vi "Actor Core.vi"(8 "error in":errorcluster, 11 "TimeTracker in":refnum<class "TimeTracker.lvclass">) -> (0 "error out":errorcluster, 3 "Actor out":refnum<class "Actor.lvclass">)   [LabVIEW 2016, in "TimeTracker.lvclass"]
doc: "(<B>Filename</B>: Actor Framework.lvlib:Actor.lvclass:Actor Core.vi)\n\nReceives messages to the actor, reacts to them, and initiates any error handling that may shut the actor down.\n\nDescendant classes may override this VI to append parallel tasks for the actor to complete while it handles messages. Overrides use the Call Parent Method node."
uses:
  TimeTracker.lvclass
  C:/Program Files (x86)/National Instruments/LabVIEW 2016/vi.lib/ActorFramework/Actor/Actor.lvclass
  <vilib>/ActorFramework/Actor/Actor.lvclass
  <vilib>/Utility/miscctls.llb/LVRectTypeDef.ctl
  DisplayWindow/DisplayWindow/DisplayWindow/DisplayWindow.lvclass
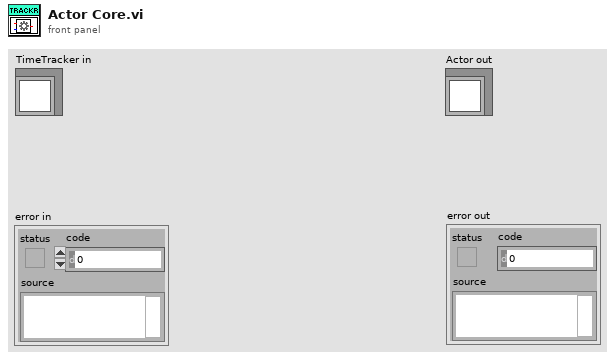
[diagram p1: front panel]
types:
  T1 = typedef "LVRectTypeDef.ctl" = cluster{"Left":i16, "Top":i16, "Right":i16, "Bottom":i16}
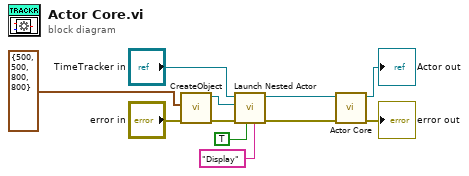
[diagram p0: block diagram]
diagram:
  n1 = call "CreateObject.vi"("error in (no error)"="error in", "Bounds"=T1 {"Left"=500, "Top"=500, "Right"=800, "Bottom"=800}) -> ("error out"=w1:errorcluster, "DisplayWindow out"=w4:refnum<class "DisplayWindow.lvclass">)  [unwired: 8 in]
  n2 = call <vilib>:"Launch Nested Actor.vi"("Debug Alias"="Display", "Open Actor Core front panel? (F)"=TRUE, "error in (no error)"=w1, "Nested Actor"=w4, "Caller Actor in"="TimeTracker in") -> ("error out"=w9:errorcluster, "Caller Actor out"=w7:refnum<class "TimeTracker.lvclass">)  [unwired: 4 in, 1 out]
  n3 = call-parent "Actor Core.vi"("error in"=w9, "Actor in"=w7) -> ("error out"=→"error out":errorcluster, "Actor out"=→"Actor out":refnum<class "Actor.lvclass">)  [unwired: 8 in]
